vi "GetDiagrams.vi"(7 "PythonConverter_BD in":refnum<class "PyConvBD.lvclass">, 8 "error in":errorcluster, 11 "Structure in":refnum<class "Structure.lvclass">) -> (0 "error out":errorcluster, 3 "Structure out":refnum<class "Structure.lvclass">, 4 "diagrams":string[](array[string]), 5 "PythonConverter_BD out":refnum<class "PyConvBD.lvclass">)   [LabVIEW 2014, in "Structure.lvclass"]
uses:
  Structure.lvclass
  Python/PythonConverter_BD/PyConvBD.lvclass
  Structure.lvclass/Structure.ctl
  Diagram/Diagram.lvclass
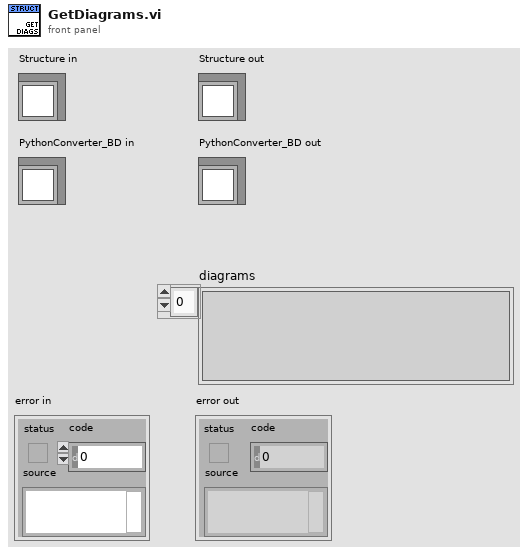
[diagram p1: front panel]
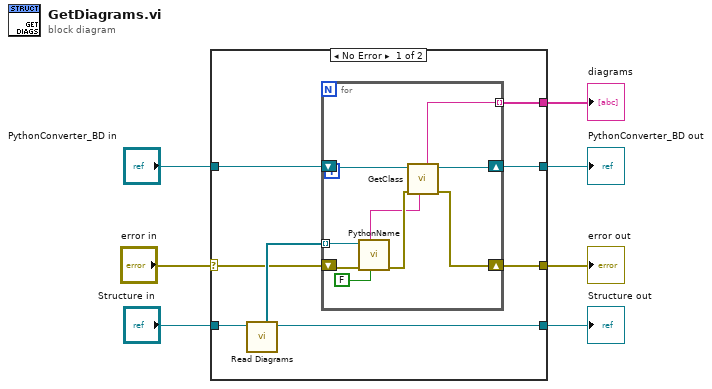
[diagram p0: block diagram]
diagram:
  n1 = case shown="No Error" "error in" {
    selector: "error in" -> [w9 w27]
    tunnel: [w11 w27] -> w6
    tunnel: [w14 w26] -> w4
    tunnel: "Structure in" -> [w15 w26]
    tunnel: [w10 w25] -> w3
    tunnel: "PythonConverter_BD in" -> [w12 w25]
    tunnel: [w8 _] -> w1
    frame No Error {
      n2 = call "Read Diagrams.vi"("Structure in"=w15) -> ("Structure out"=w14:refnum<class "Structure.lvclass">, "Diagrams"=w13:refnum<class "Diagram.lvclass">[])  [unwired: 7 in]
      n3 = for {
        tunnel: w13 -> [w24] mode=indexing
        shift-right: [w22] -> w10
        shift-left: w12 -> [w23]
        shift-right: [w19] -> w11
        shift-left: w9 -> [w20]
        tunnel: [w18] -> w8 mode=indexing
        n4 = call-dynamic "PythonName.vi"("add self"=FALSE, "error in"=w20, "Diagram in"=w24) -> ("error out"=w21:errorcluster, "UID"=w16:string)  [unwired: 5 in, 2 out]
        n5 = call "GetClass.vi"("name"=w16, "error in"=w21, "PythonConverter_BD in"=w23) -> ("error out"=w19:errorcluster, "PythonConverter_BD out"=w22:refnum<class "PyConvBD.lvclass">, "class"=w18:string)  [unwired: 4 in]
      }
    }
    frame Error {
    }
  }
  "error out" <- w6
  "Structure out" <- w4
  "PythonConverter_BD out" <- w3
  "diagrams" <- w1
